vi "Interface.vi"(9 "EventsIn":T1, 10 "Events":T2) -> ()   [LabVIEW 2014, in "GCMIconEditor.lvlib" / "GCMIconEditor.lvclass"]
uses:
  GCMIconEditor.lvclass
  Framework/_Plugins/_LVCMPlugin/GCMPlugin_EventsOut.ctl
  Framework/_Plugins/_LVCMPlugin/GCMPlugin_EventsIn.ctl
  <vilib>/LabVIEW Icon API/lv_icon/Classes/Icon/Icon.lvclass
  Command.ctl
  <vilib>/LabVIEW Icon API/API_Text.ctl
  <vilib>/LabVIEW Icon API/API_Test Settings.ctl
  <vilib>/LabVIEW Icon API/lv_icon/Controls/Alignment.ctl
  <vilib>/LabVIEW Icon API/API_Text Colors.ctl
  <vilib>/LabVIEW Icon API/lv_icon/Controls/Layer.ctl
  <vilib>/LabVIEW Icon API/lv_icon/Controls/LayerType.ctl
  <vilib>/Utility/miscctls.llb/LVPoint32TypeDef.ctl
  <vilib>/LabVIEW Icon API/lv_icon/Classes/Layer/Layer.lvclass
  <vilib>/LabVIEW Icon API/lv_icon/Classes/Icon Framework/Icon Framework.lvclass
  <vilib>/LabVIEW Icon API/LabVIEW Icon API.lvlib
  Framework/_Plugins/GCMPlugin/GCMPlugin.lvclass
panel:
  in  "LoadDefaultFontSettings":bool
  in  "Capitalize text":bool
  in  "Center text vertically":bool
  in  "Alignment":u16(ring) caption="Ring" items=["left", "center", "right"]
  in  "Font Size":u8
  in  "Line 4 Color":u32(colorbox)
  in  "Line 3 Color":u32(colorbox)
  in  "Line 2 Color":u32(colorbox)
  in  "Line 1 Color":u32(colorbox) caption="Text Color"
  in  "Line 4":string
  in  "Line 3":string
  in  "Line 2":string
  in  "Line 1":string
  in  "ClearIcon":bool
  in  "RemoveNIIconNumber":bool
  out "Zoomed Icon":picture
  out "Icon":picture
  # "Icon Text"
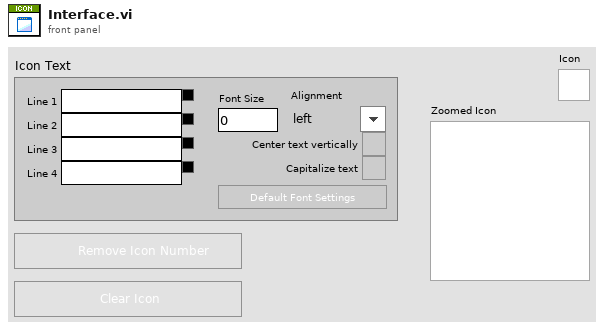
[diagram p1: front panel]
types:
  T1 = typedef "GCMPlugin.lvclass/GCMPlugin_EventsIn.ctl" = cluster{"Stop":refnum<user-event>, "ItemSelected":refnum<user-event>, "ItemDeselected":refnum<user-event>, "PluginActivated":refnum<user-event>, "PluginDeactivated":refnum<user-event>}
  T2 = typedef "GCMPlugin.lvclass/GCMPlugin_EventsOut.ctl" = cluster{"ItemEdited":refnum<user-event>}
  T3 = typedef "GCMIconEditor.lvlib/GCMIconEditor.lvclass/Command.ctl" = enum16{"ShowIcon", "ApplyIconToVI"}
  T4 = typedef "LabVIEW Icon API.lvlib/API_Test Settings.ctl" = cluster{"Font":string, "Alignment":T5, "Size":u8, "Center text":bool, "Capitalize text":bool, "Text color":T6}
  T5 = typedef "Alignment.ctl" = u16
  T6 = typedef "LabVIEW Icon API.lvlib/API_Text Colors.ctl" = cluster{"Line 1 color":u32, "Line 2 color":u32, "Line 3 color":u32, "Line 4 color":u32}
  T7 = typedef "LabVIEW Icon API.lvlib/API_Text.ctl" = cluster{"Line 1 text":string, "Line 2 text":string, "Line 3 text":string, "Line 4 text":string}
  T8 = typedef "LVPoint32TypeDef.ctl" = cluster{"Horizontal":i32, "Vertical":i32}
  T9 = typedef "LayerType.ctl" = enum16{"Graphic", "Text", "Tool", "Graphic Drop"}
  T10 = cluster{"left":i16, "top":i16, "right":i16, "bottom":i16}
  T11 = typedef "Layer.ctl" = cluster{"LayerIcon":picture, "LayerName":string, "Opacity":u8, "Visibility?":bool}
  T12 = typedef "BodyText.ctl" = cluster{"Line 1 text":string, "Line 2 text":string, "Line 3 text":string, "Line 4 text":string, "Line 1 color":u32, "Line 2 color":u32, "Line 3 color":u32, "Line 4 color":u32, "Body Text Spec":cluster{"Font":T13, "Alignment":T5, "Size":u8}, "Center text vertically":bool, "Capitalize Text":bool}
  T13 = typedef "Font.ctl" = string
  T14 = typedef "imagedata.ctl" = cluster{"image type":i32, "image depth":i32, "image":u8[], "mask":u8[], "colors":u32[], "Rectangle":cluster{"left":i16, "top":i16, "right":i16, "bottom":i16}}
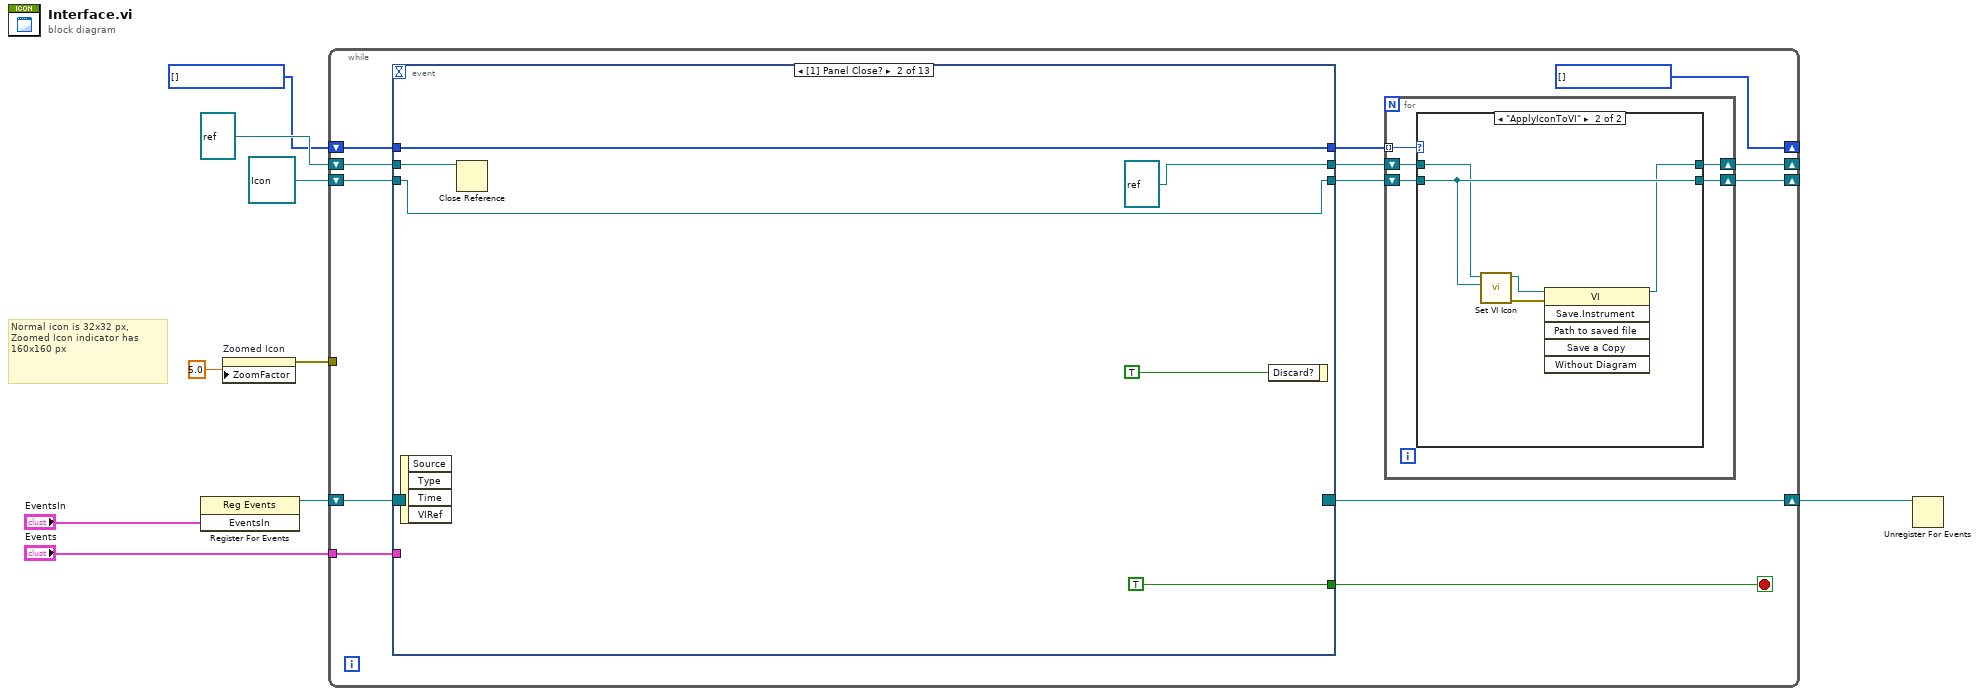
[diagram p0: block diagram]
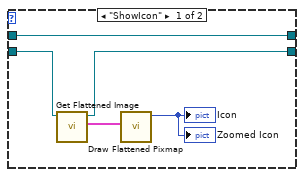
[diagram p2: hidden frame]
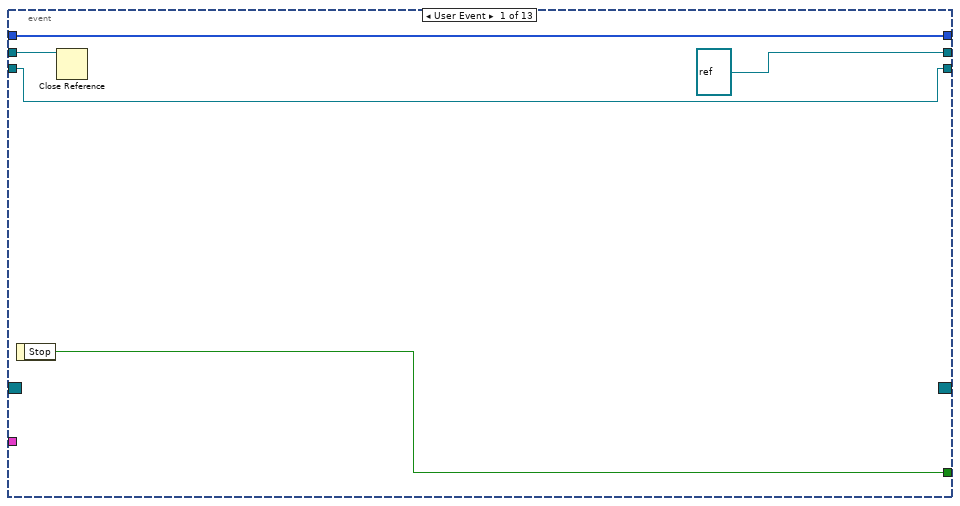
[diagram p3: hidden frame]
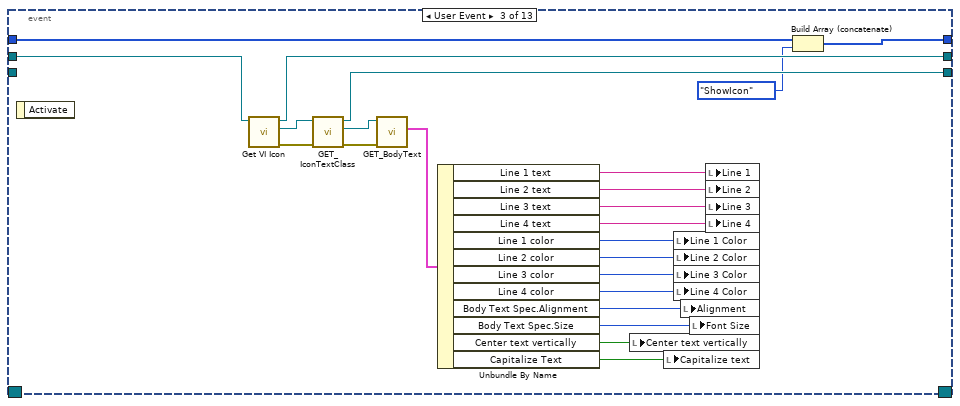
[diagram p4: hidden frame]
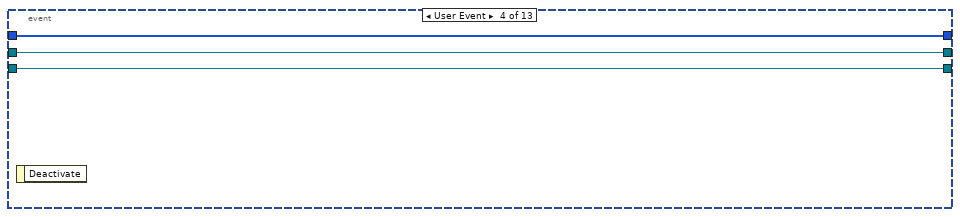
[diagram p5: hidden frame]
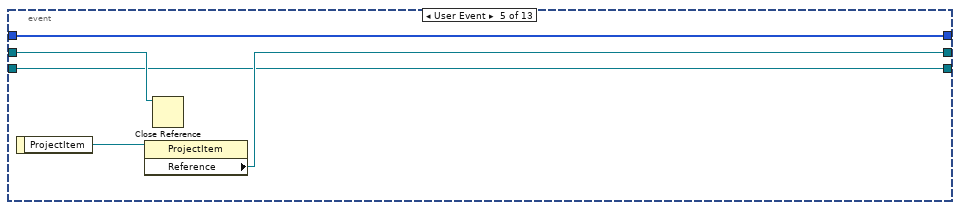
[diagram p6: hidden frame]
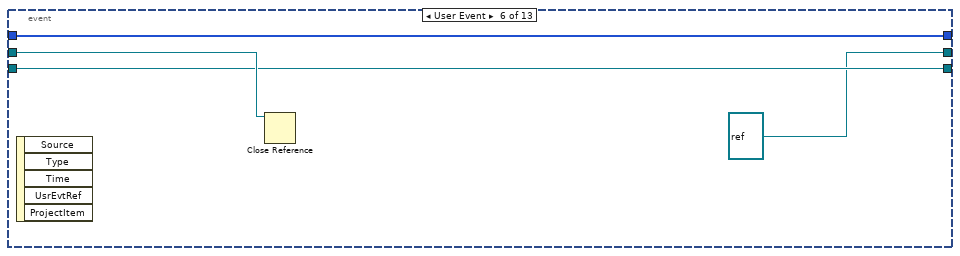
[diagram p7: hidden frame]
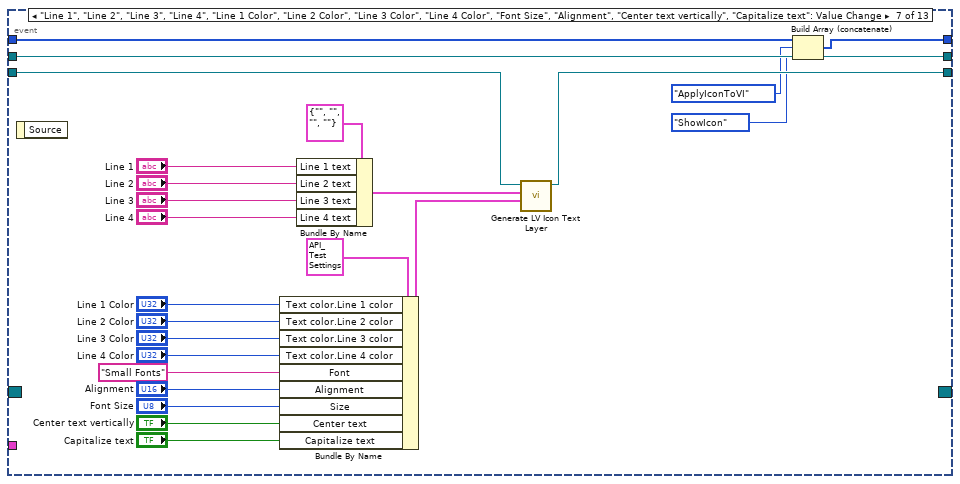
[diagram p8: hidden frame]
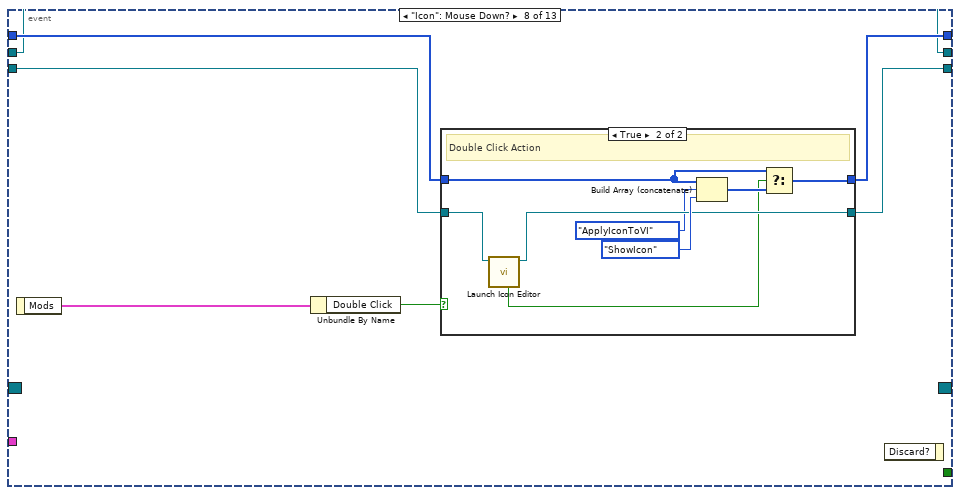
[diagram p9: hidden frame]
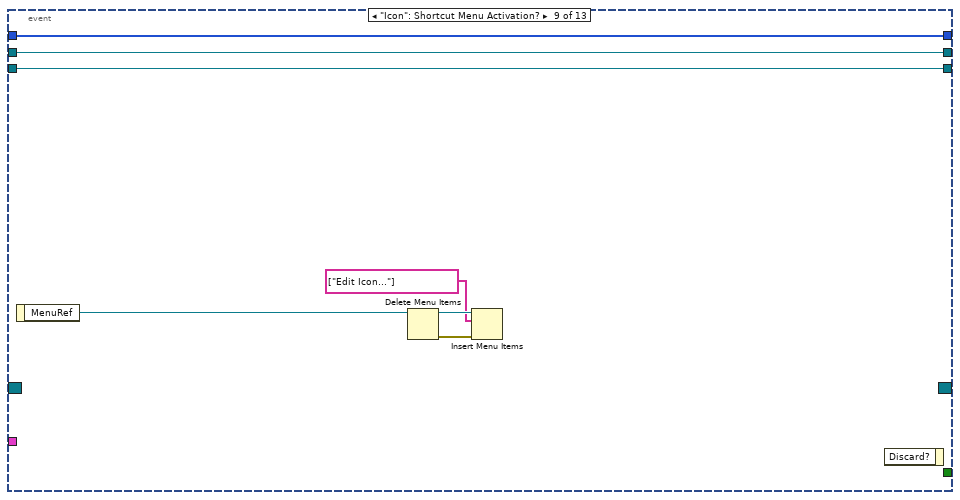
[diagram p11: hidden frame]
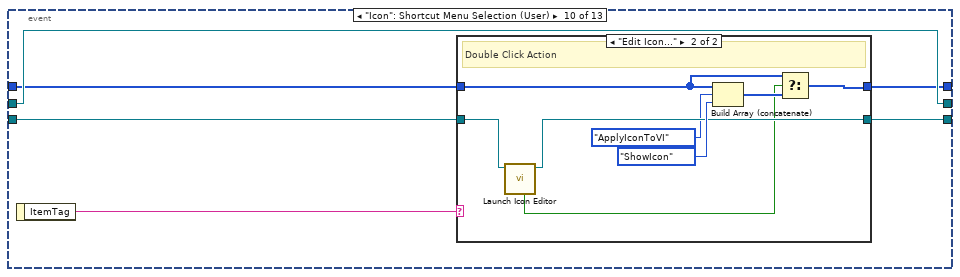
[diagram p12: hidden frame]
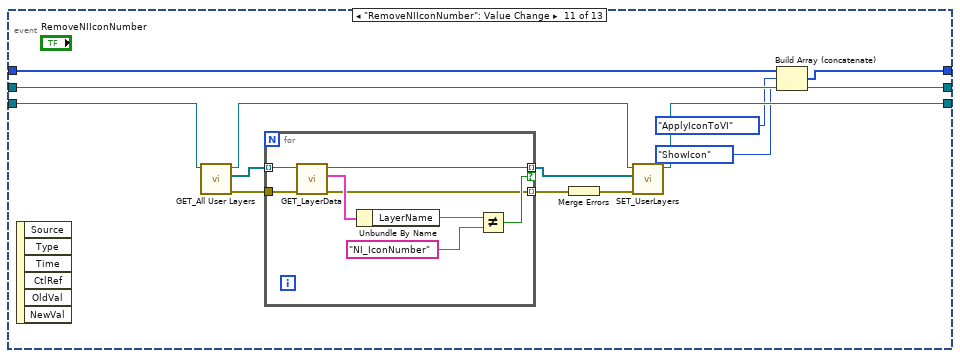
[diagram p14: hidden frame]
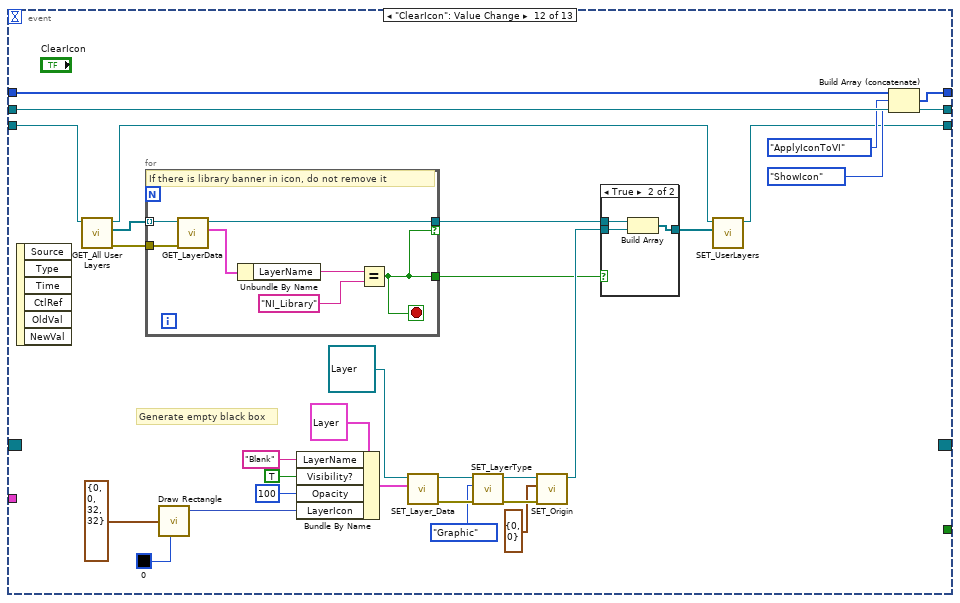
[diagram p15: hidden frame]
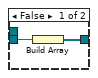
[diagram p16: hidden frame]
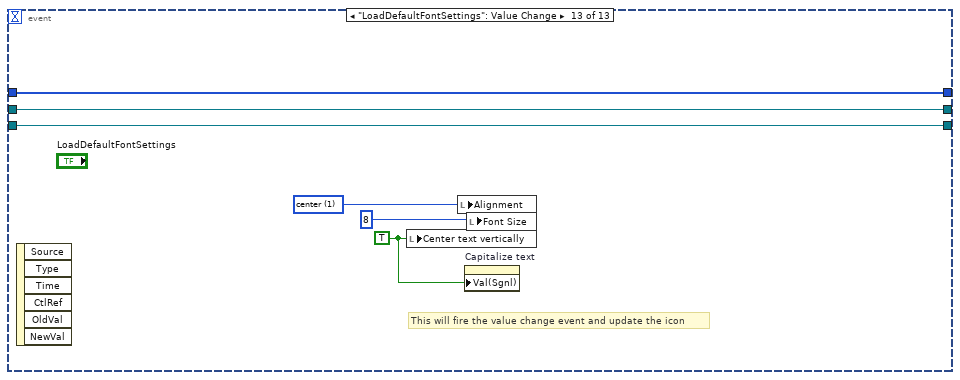
[diagram p17: hidden frame]
diagram:
  w1 = T3[] [] items=["ShowIcon", "ApplyIconToVI"]
  # "Normal icon is 32x32 px, Zoomed Icon indicator has 160x160 px"
  n1 = register-events("EventsIn") -> (reference out=w8:refnum<event-registration>)  [unwired: 2 in, 1 out]
  n2 = property on="Zoomed Icon" class="Pict"("ZoomFactor"=sgl 5.0 ("Zoom Factor")) -> (error out=w2:errorcluster)  [unwired: 2 in, 1 out]
  n3 = while {
    tunnel: "Events" -> [w21]
    shift-right: [w18] -> w6
    shift-left: w8 -> [w22]
    shift-right: [w13] -> _
    shift-left: refnum<vi> refnum ("VI Refnum out") -> [w19]
    shift-right: [w11] -> _
    shift-left: refnum<class "Icon.lvclass"> refnum ("lv_icon.lvlib:Icon.lvclass out") -> [w17]
    tunnel: w2 -> [_]
    shift-right: [w10] -> _
    shift-left: w1 -> [w16]
    stop <- w20 stop-if-true
    w10 = T3[] [] items=["ShowIcon", "ApplyIconToVI"]
    n4 = event shown="[1] Panel Close?" {
      selector: w22 -> [_ _ _ _ _ _ _ _ _ _ _ _ _]
      dyn-events: [_ _ _ _ _ _ _ _ _ _ _ _ _] -> w18
      timeout: _ -> [_ _ _ _ _ _ _ _ _ _ _ _ _]
      tunnel: w21 -> [_ _ _ _ _ _ _ _ _ _ _ _ _]
      tunnel: [w42 TRUE ("Stop") _ _ _ _ _ _ _ _ _ _ _] -> w20
      tunnel: w19 -> [w41 w46 w49 w73 w76 w82 w107 w108 w127 w137 w153 w197 w210]
      tunnel: [refnum<vi> refnum ("VI Refnum out") refnum<vi> refnum ("VI Refnum out") w71 w73 w77 refnum<vi> refnum ("VI Refnum out") w107 w108 w127 w137 w153 w197 w210] -> w14
      tunnel: [w39 w44 w67 w72 w75 w81 w88 w110 w126 w133 w152 w176 w215] -> w12
      tunnel: w17 -> [w39 w44 _ w72 w75 w81 w106 w109 w126 w134 w159 w190 w215]
      tunnel: w16 -> [w38 w43 w52 w74 w79 w83 w87 w112 w125 w136 w149 w194 w214]
      tunnel: [w38 w43 w51 w74 w79 w83 w86 w111 w125 w135 w148 w193 w214] -> w15
      event User Event {
        n5 = event-data() -> ("Stop"=w42:bool)  [unwired: 1 in]
        n6 = Close Reference(reference=w41) -> ()  [unwired: 1 in, 1 out]
      }
      event Panel Close? {
        n7 = event-data() -> ()  [unwired: 1 in, 4 out]
        n8 = Close Reference(reference=w46) -> ()  [unwired: 1 in, 1 out]
        n9 = event-data("Discard?"=TRUE) -> ()  [unwired: 1 in, 1 out]
      }
      event User Event {
        n10 = event-data() -> ()  [unwired: 1 in, 1 out]
        n11 = call <vilib>:"Get VI Icon.vi"("VI Refnum in"=w49) -> ("error out"=w69:errorcluster, "Icon"=w53:refnum<class "Icon.lvclass">, "VI Refnum out"=w71:refnum<vi>)  [unwired: 8 in]
        n12 = call-dynamic "GET_IconTextClass.vi"("error in (no error)"=w69, "Icon.lvclass in"=w53) -> ("error out"=w68:errorcluster, "Icon Framework.lvclass"=w70:refnum<class "Icon Framework.lvclass">, "Icon.lvclass out"=w67:refnum<class "Icon.lvclass">)  [unwired: 7 in]
        n13 = call-dynamic "GET_BodyText.vi"("error in (no error)"=w68, "Icon Framework.lvclass in"=w70) -> ("Body Text"=w66:T12)  [unwired: 6 in, 3 out]
        n14 = Unbundle By Name(w66) -> ("Line 1 text"=w65:string, "Line 2 text"=w64:string, "Line 3 text"=w63:string, "Line 4 text"=w62:string, "Line 1 color"=w61:u32, "Line 2 color"=w60:u32, "Line 3 color"=w59:u32, "Line 4 color"=w58:u32, "Body Text Spec.Alignment"=w57:T5, "Body Text Spec.Size"=w56:u8, "Center text vertically"=w55:bool, "Capitalize Text"=w54:bool)
        n15 = local write "Center text vertically"(w55) -> ()
        n16 = local write "Capitalize text"(w54) -> ()
        n17 = local write "Line 1 Color"(w61) -> ()
        n18 = local write "Line 2 Color"(w60) -> ()
        n19 = local write "Line 3 Color"(w59) -> ()
        n20 = local write "Line 4 Color"(w58) -> ()
        n21 = local write "Alignment"(w57) -> ()
        n22 = local write "Font Size"(w56) -> ()
        n23 = local write "Line 1"(w65) -> ()
        n24 = local write "Line 2"(w64) -> ()
        n25 = local write "Line 3"(w63) -> ()
        n26 = local write "Line 4"(w62) -> ()
        n27 = Build Array (concatenate)(w52, Command."ShowIcon" ("Command")) -> (w51:T3[])
      }
      event User Event {
        n28 = event-data() -> ()  [unwired: 1 in, 1 out]
      }
      event User Event {
        n29 = event-data() -> ("ProjectItem"=w78:refnum<vi>)  [unwired: 1 in]
        n30 = property class="ProjectItem"(reference=w78) -> ("Reference"=w77:refnum<vi>)  [unwired: 1 in, 2 out]
        n31 = Close Reference(reference=w76) -> ()  [unwired: 1 in, 1 out]
      }
      event User Event {
        n32 = event-data() -> ()  [unwired: 1 in, 5 out]
        n33 = Close Reference(reference=w82) -> ()  [unwired: 1 in, 1 out]
      }
      event "Line 1", "Line 2", "Line 3", "Line 4", "Line 1 Color", "Line 2 Color", "Line 3 Color", "Line 4 Color", "Font Size", "Alignment", "Center text vertically", "Capitalize text": Value Change {
        n34 = event-data() -> ()  [unwired: 1 in, 1 out]
        n35 = Bundle By Name(cluster=T4 {"Font"="Small Fonts", "Alignment"=1, "Size"=8, "Center text"=TRUE, "Capitalize text"=TRUE, "Text color"={"Line 1 color"=0, "Line 2 color"=0, "Line 3 color"=0, "Line 4 color"=0}} ("Text settings"), "Text color.Line 1 color"="Line 1 Color", "Text color.Line 2 color"="Line 2 Color", "Text color.Line 3 color"="Line 3 Color", "Text color.Line 4 color"="Line 4 Color", "Font"="Small Fonts", "Alignment"="Alignment", "Size"="Font Size", "Center text"="Center text vertically", "Capitalize text"="Capitalize text") -> (w89:T4)
        n36 = Bundle By Name(cluster=T7 {"Line 1 text"="", "Line 2 text"="", "Line 3 text"="", "Line 4 text"=""} ("Text"), "Line 1 text"="Line 1", "Line 2 text"="Line 2", "Line 3 text"="Line 3", "Line 4 text"="Line 4") -> (w100:T7)
        n37 = call <vilib>:"Generate LV Icon Text Layer.vi"("Text settings"=w89, "Text"=w100, "Icon in"=w106) -> ("Icon out"=w88:refnum<class "Icon.lvclass">)  [unwired: 7 in, 1 out]
        n38 = Build Array (concatenate)(w87, Command."ApplyIconToVI" ("Command"), Command."ShowIcon" ("Command")) -> (w86:T3[])
      }
      event "Icon": Mouse Down? {
        n39 = event-data() -> ("Mods"=w114:cluster{"Double Click":bool, "Menu Key":bool})  [unwired: 1 in]
        n40 = Unbundle By Name(w114) -> ("Double Click"=w113:bool)
        n41 = case shown="True" w113 {
          tunnel: w112 -> [w116 w117]
          tunnel: [w116 w119] -> w111
          tunnel: [w115 w122] -> w110
          tunnel: w109 -> [w115 w123]
          frame False {
            # "Single Click Action"
          }
          frame True {
            # "Double Click Action"
            n42 = call <vilib>:"Launch Icon Editor.vi"("Icon in"=w123) -> ("Icon out"=w122:refnum<class "Icon.lvclass">, "Canceled?"=w118:bool)  [unwired: 8 in, 1 out]
            n43 = Build Array (concatenate)(w117, Command."ApplyIconToVI" ("element"), Command."ShowIcon" ("Command")) -> (w120:T3[])
            n44 = Select(t=w117, s=w118, f=w120) -> (s? t:f=w119:T3[])
          }
        }
        n45 = event-data() -> ()  [unwired: 2 in, 1 out]
      }
      event "Icon": Shortcut Menu Activation? {
        n46 = event-data() -> ("MenuRef"=w131:refnum<k9>)  [unwired: 1 in]
        n47 = Delete Menu Items(9:w131) -> (0:w129:errorcluster, 3:w130:refnum<k9>)  [unwired: 3 in]
        n48 = Insert Menu Items(6:w129, 8:string[] ["Edit Icon..."] ("item names"), 9:w130) -> ()  [unwired: 3 in, 3 out]
        n49 = event-data() -> ()  [unwired: 2 in, 1 out]
      }
      event "Icon": Shortcut Menu Selection (User) {
        n50 = event-data() -> ("ItemTag"=w132:string)  [unwired: 1 in]
        n51 = case shown="\"Edit Icon...\"" w132 {
          tunnel: w136 -> [w139 w140]
          tunnel: [w139 w142] -> w135
          tunnel: [w138 w145] -> w133
          tunnel: w134 -> [w138 w146]
          frame Default {
            # "Single Click Action"
          }
          frame "Edit Icon..." {
            # "Double Click Action"
            n52 = call <vilib>:"Launch Icon Editor.vi"("Icon in"=w146) -> ("Icon out"=w145:refnum<class "Icon.lvclass">, "Canceled?"=w141:bool)  [unwired: 8 in, 1 out]
            n53 = Build Array (concatenate)(w140, Command."ApplyIconToVI" ("element"), Command."ShowIcon" ("Command")) -> (w143:T3[])
            n54 = Select(t=w140, s=w141, f=w143) -> (s? t:f=w142:T3[])
          }
        }
      }
      event "RemoveNIIconNumber": Value Change {
        n55 = event-data() -> ()  [unwired: 1 in, 6 out]
        n56 = call-dynamic "GET_All User Layers.vi"("Icon.lvclass in"=w159) -> ("error out"=w158:errorcluster, "User Layer"=w160:refnum<class "Layer.lvclass">[], "Icon.lvclass out"=w154:refnum<class "Icon.lvclass">)  [unwired: 8 in]
        n57 = for {
          tunnel: w160 -> [w168] mode=indexing
          tunnel: w158 -> [w167]
          tunnel: [w163] -> w155 mode=indexing if=w162
          tunnel: [w161] -> w157 mode=indexing
          n58 = call-dynamic "GET_LayerData.vi"("error in (no error)"=w167, "Layer.lvclass in"=w168) -> ("error out"=w161:errorcluster, "Data"=w166:T11, "Layer.lvclass out"=w163:refnum<class "Layer.lvclass">)  [unwired: 5 in, 2 out]
          n59 = Unbundle By Name(w166) -> ("LayerName"=w165:string)
          n60 = Not Equal?(x=w165, y="NI_IconNumber") -> (x != y?=w162:bool)
        }
        n61 = Merge Errors(w157) -> (w156:errorcluster)
        n62 = call-dynamic "SET_UserLayers.vi"("error in (no error)"=w156, "Layers"=w155, "Icon.lvclass in"=w154) -> ("Icon.lvclass out"=w152:refnum<class "Icon.lvclass">)  [unwired: 7 in, 1 out]
        n63 = Build Array (concatenate)(w149, Command."ApplyIconToVI" ("Command"), Command."ShowIcon" ("Command")) -> (w148:T3[])
      }
      event "ClearIcon": Value Change {
        # "Generate empty black box"
        n64 = event-data() -> ()  [unwired: 1 in, 6 out]
        n65 = call-dynamic "GET_All User Layers.vi"("Icon.lvclass in"=w190) -> ("error out"=w191:errorcluster, "User Layer"=w192:refnum<class "Layer.lvclass">[], "Icon.lvclass out"=w177:refnum<class "Icon.lvclass">)  [unwired: 8 in]
        n66 = for {
          tunnel: w192 -> [w209] mode=indexing
          tunnel: w191 -> [w208]
          tunnel: [w204] -> w171 if=w203
          tunnel: [w203] -> w170
          stop <- w203 stop-if-true
          # "If there is library banner in icon, do not remove it"
          n67 = call-dynamic "GET_LayerData.vi"("error in (no error)"=w208, "Layer.lvclass in"=w209) -> ("Data"=w205:T11, "Layer.lvclass out"=w204:refnum<class "Layer.lvclass">)  [unwired: 5 in, 3 out]
          n68 = Unbundle By Name(w205) -> ("LayerName"=w207:string)
          n69 = Equal?(x=w207, y="NI_Library") -> (x = y?=w203:bool)
        }
        n70 = call <vilib>:"Draw Rectangle.vi"("rect"=T10 {"left"=0, "top"=0, "right"=32, "bottom"=32}, "color(black)"=u32 0) -> ("new picture"=w186:picture)  [unwired: 7 in]
        n71 = Bundle By Name(cluster=T11 {"LayerIcon"=bytes[0], "LayerName"="", "Opacity"=0, "Visibility?"=FALSE} ("Data"), "LayerName"="Blank", "Visibility?"=TRUE, "Opacity"=u8 100, "LayerIcon"=w186) -> (w175:T11)
        n72 = call-dynamic "SET_Layer_Data.vi"("Data"=w175, "Layer.lvclass in"=refnum<class "Layer.lvclass"> refnum) -> ("error out"=w182:errorcluster, "Layer.lvclass out"=w181:refnum<class "Layer.lvclass">)  [unwired: 2 in, 6 out]
        n73 = call-dynamic "SET_LayerType.vi"("error in (no error)"=w182, "Type"=LayerType."Graphic", "Layer.lvclass in"=w181) -> ("error out"=w178:errorcluster, "Layer.lvclass out"=w179:refnum<class "Layer.lvclass">)  [unwired: 7 out]
        n74 = call-dynamic "SET_Origin.vi"("error in (no error)"=w178, "Point32"=T8 {"Horizontal"=0, "Vertical"=0}, "Layer.lvclass in"=w179) -> ("Layer.lvclass out"=w173:refnum<class "Layer.lvclass">)  [unwired: 7 in, 1 out]
        n75 = case shown="True" w170 {
          tunnel: w173 -> [w199 w202]
          tunnel: [w198 w201] -> w172
          tunnel: w171 -> [_ w200]
          frame False {
            n76 = Build Array(w199) -> (w198:refnum<class "Layer.lvclass">[])
          }
          frame True {
            n77 = Build Array(w200, w202) -> (w201:refnum<class "Layer.lvclass">[])
          }
        }
        n78 = call-dynamic "SET_UserLayers.vi"("Layers"=w172, "Icon.lvclass in"=w177) -> ("Icon.lvclass out"=w176:refnum<class "Icon.lvclass">)  [unwired: 8 in, 1 out]
        n79 = Build Array (concatenate)(w194, Command."ApplyIconToVI" ("Command"), Command."ShowIcon" ("Command")) -> (w193:T3[])
      }
      event "LoadDefaultFontSettings": Value Change {
        w211 = TRUE ("Center text vertically")
        w213 = u16 1 items=["left", "center", "right"] ("Alignment")
        # "This will fire the value change event and update the icon"
        n80 = event-data() -> ()  [unwired: 1 in, 6 out]
        n81 = local write "Center text vertically"(w211) -> ()
        n82 = local write "Alignment"(w213) -> ()
        n83 = property on="Capitalize text" class="Bool (strict)"("Val(Sgnl)"=w211) -> ()  [unwired: 2 in, 2 out]
        n84 = local write "Font Size"(u8 8 ("Font Size")) -> ()
      }
    }
    n85 = for {
      tunnel: w15 -> [w27] mode=indexing
      shift-right: [w25] -> w13
      shift-left: w14 -> [w26]
      shift-right: [w24] -> w11
      shift-left: w12 -> [w23]
      n86 = case shown="\"ApplyIconToVI\"" w27 {
        tunnel: w26 -> [w32 w34]
        tunnel: [w32 w33] -> w25
        tunnel: [w28 w35] -> w24
        tunnel: w23 -> [w29 w35]
        frame "ShowIcon" {
          n87 = call <vilib>:"Get Flattened Image.vi"("lv_icon.lvlib:Icon.lvclass in"=w29) -> ("Color Image"=w31:T14, "lv_icon.lvlib:Icon.lvclass out"=w28:refnum<class "Icon.lvclass">)  [unwired: 7 in, 2 out]
          n88 = call <vilib>:"Draw Flattened Pixmap.vi"("image data"=w31) -> ("new picture"=→"Icon" →"Zoomed Icon":picture)  [unwired: 8 in]
        }
        frame "ApplyIconToVI" {
          n89 = call <vilib>:"Set VI Icon.vi"("Icon"=w35, "VI Refnum in"=w34) -> ("error out"=w36:errorcluster, "VI Refnum out"=w37:refnum<vi>)  [unwired: 8 in]
          n90 = invoke class="VI" method="Save.Instrument"(reference=w37, error in=w36) -> (reference out=w33:refnum<vi>)  [unwired: 4 in, 5 out]
        }
      }
    }
  }
  n91 = Unregister For Events(event registration refnum=w6) -> ()  [unwired: 1 in, 1 out]
